vi "get_component_type_name.vi"(8 "error in (no error)":errorcluster, 11 "GenericPlugin in":refnum<class "GenericFPGAWrapper.lvclass">) -> (0 "error out":errorcluster, 2 "component type":string, 3 "GenericPlugin out":refnum<class "GenericFPGAWrapper.lvclass">)   [LabVIEW 2010, in "GenericFPGAWrapper.lvclass"]
uses:
  GenericFPGAWrapper.lvclass
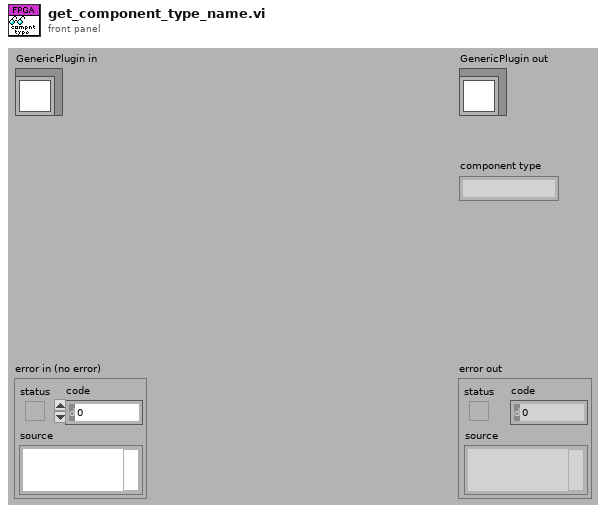
[diagram p1: front panel]
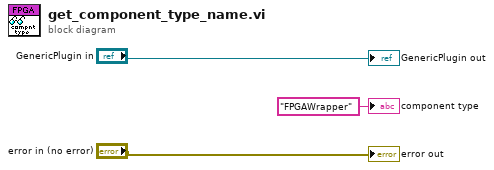
[diagram p0: block diagram]
diagram:
  "error out" <- "error in (no error)"
  "GenericPlugin out" <- "GenericPlugin in"
  "component type" <- "FPGAWrapper" ("component type")
